vi "Get Diagnostic Value.vi"(0 "VISA Session In":refnum<visa-resource-name>="OXYMAT", 1 "Target Address":u8=16 format="%.0x", 2 "Source Address":u8=208 format="%.0x", 7 "Diagnostic Value":T1(ring)=enum."Temperature of physical section", 11 "error in (no error)":errorcluster) -> (4 "VISA Session Out":refnum<visa-resource-name>, 6 "Message Header":T3 {"Source Address" format="%.0x"; "Target Address" format="%.0x"}, 10 "Measurement":cluster{"Measured value":dbl, "Dimension":T2}={"Measured value"=nan, "Dimension"=enum."Unknown (0)"} {"Measured value" format="%#_6f"}, 13 "Success":bool, 15 "error out":errorcluster)   [LabVIEW 2019, in "Siemens ELAN.lvlib"]
doc: "Using the Siemens ELAN protocol, gets the specified diagnostic value from the analyzer. Returns measured real value and unit of measure. Also returns a boolean indicating that the addressed device provided a valid response.\n\n$Revision:: 0 $\n$Modtime:: yy-mm-dd hh:mm $\n$Author:: Dboyd $"
uses:
  Siemens ELAN.lvlib
  Unit Dimensions.ctl
  Message Header.ctl
  Channel Status.ctl
panel:
  in  "Dimension":T2
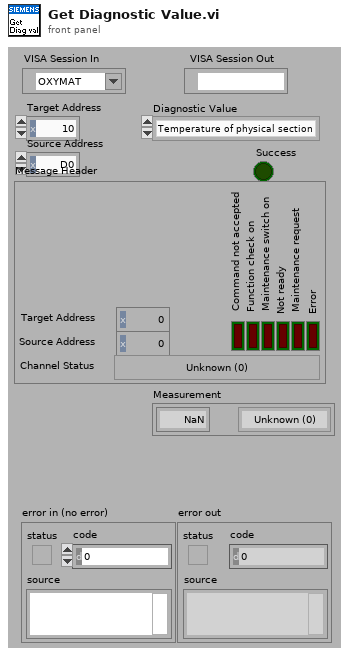
[diagram p1: front panel]
types:
  T1 = enum8{"Unused (0)", "Temperature of physical section", "Temperature of measuring head", "Detector raw signal", "Magnetic field", "Temperature of display", "Calibration reserve", "Analog input", "Signal vector", "Disturbance vector", "Unused (>9)"}
  T2 = typedef "Siemens ELAN.lvlib/Unit Dimensions.ctl" = enum8{"Unknown (0)", "Pure number", "ppm", "ppb", "vpm", "vpm C1", "vpm C3", "vpm C6", "mg C/m^3", "mg/m^3", "%", "% v/v", "% of range", "% saturation", "%/°C", "%/K", "% w/w", "mV/pH", "mV/mbar", "nA/mbar", "S/m", "S/cm", "mS/m", "mS/cm", "uS/m", "uS/cm", "s", "min", "hr", "pA", "mA", "uV", "mV", "V", "mbar", "hPa", "ml/min", "kohm", "MOhm", "S", "°C", "Hz", "pH", "ug/l", "mg/l", "l/min", "uA", "mg/dm^3", "kPa", "kohm*cm", "MOhm*cm", "°", "Unknown (>51)"}
  T3 = typedef "Siemens ELAN.lvlib/Message Header.ctl" = cluster{"Target Address":u8, "Source Address":u8, "Error":bool, "Maintenance request":bool, "Not ready":bool, "Maintenance switch on":bool, "Function check on":bool, "Command not accepted":bool, "Channel Status":T4}
  T4 = typedef "Siemens ELAN.lvlib/Channel Status.ctl" = enum8{"Unknown (0)", "Warm-up", "Pause", "Standby", "Measure", "Zero calibration", "Adjust component slope", "Unknown (7)", "Adjust curve dip", "Adjust linearization sensitivity", "Adjust temperature compensation", "Adjust pressure compensation", "Adjust linearization zero", "Adjust flow sensor", "Autocal", "Adjust phase", "Zero calibration of O2 sensor", "Synchronous zero calibration", "Purging for synchronous zero calibration", "Adjust analog output", "Adjust analog input", "Cleaning", "Unknown (>21)"}
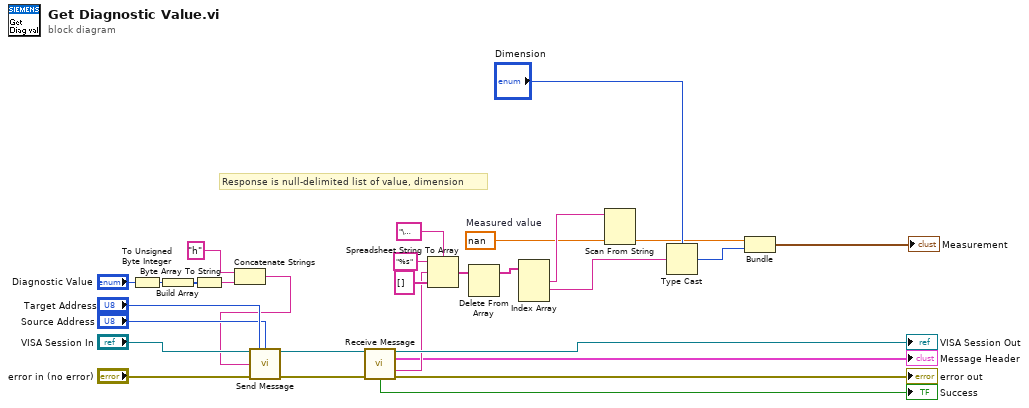
[diagram p0: block diagram]
diagram:
  w12 = nan  # Measured value
  # "Response is null-delimited list of value, dimension"
  n1 = To Unsigned Byte Integer(number="Diagnostic Value") -> (unsigned 8bit integer=w5:u8)
  n2 = Build Array(w5) -> (w4:u8[])
  n3 = Byte Array To String(unsigned byte array=w4) -> (string=w3:string)
  n4 = Concatenate Strings("h" ("Command"), w3) -> (w1:string)
  n5 = call "Send Message.vi"("VISA Session In"="VISA Session In", "Target Address"="Target Address", "Source Address"="Source Address", "Command"=w1, "error in (no error)"="error in (no error)") -> ("VISA Session Out"=w29:refnum<visa-resource-name>, "error out"=w28:errorcluster)  [unwired: 8 in, 1 out]
  n6 = call "Receive Message.vi"("VISA Session In"=w29, "error in (no error)"=w28) -> ("VISA Session Out"=→"VISA Session Out":refnum<visa-resource-name>, "Message Header"=→"Message Header":T3, "Response"=w19:string, "Success"=→"Success":bool, "error out"=→"error out":errorcluster)  [unwired: 8 in, 1 out]
  n7 = Spreadsheet String To Array(delimiter (Tab)="\u0000", format string="%s", spreadsheet string=w19, array type (2D Dbl)=string[] []) -> (array=w16:string[])
  n8 = Delete From Array(array=w16) -> (array with subset deleted=w15:string[])  [unwired: 2 in, 1 out]
  n9 = Index Array(array=w15) -> (element #1=w13:string, element #2=w7:string)  [unwired: 3 in, 1 out]
  n10 = Scan From String(input string=w13, default 1=w12) -> (output 1=w9:dbl)  [unwired: 3 in, 3 out]
  n11 = Type Cast(type="Dimension", x=w7) -> (*(type *) &x=w8:T2)
  n12 = Bundle("Measured value"=w9, "Dimension"=w8) -> (→"Measurement":cluster{"Measured value":dbl, "Dimension":T2})  [unwired: 1 in]
